vi "sort channels for specific data types.vi"(8 "error in (no error)":errorcluster, 10 "data types":T1[](array[typedef]), 11 "channels in":refnum<class "TBM channel.lvclass">[](array[class])) -> (0 "error out":errorcluster, 3 "channels out":refnum<class "TBM channel.lvclass">[](array[class]))   [LabVIEW 2014, in "Shared Memory configuration.lvclass"]
uses:
  Shared Memory configuration.lvclass
  <vilib>/NI/Tag Bus/tag/Data Type.ctl
  <vilib>/NI/Tag Bus Module Framework/channel/TBM channel.lvclass
  <vilib>/NI/Tag Bus Module Framework/channel/channel classification.ctl
  <vilib>/NI/Tag Bus/tag/tag descriptor.lvclass
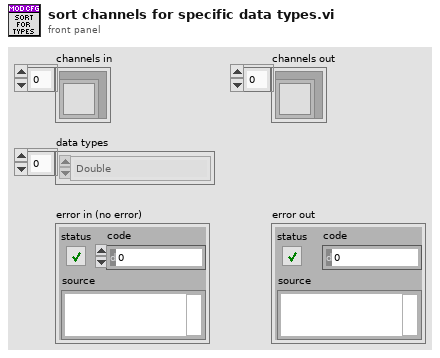
[diagram p1: front panel]
types:
  T1 = typedef "tag bus.lvlib/tag descriptor.lvclass/Data Type.ctl" = enum16{"Double", "Single", "I64", "I32", "I16", "I8", "U64", "U32", "U16", "U8", "Boolean", "String", "Array of Double", "Array of Single", "Array of I64", "Array of I32", "Array of I16", "Array of I8", "Array of U64", "Array of U32", "Array of U16", "Array of U8", "Array of Boolean", "Array of String"}
  T2 = typedef "TBM channel.lvclass/channel classification.ctl" = enum16{"input data", "output data", "processing parameter", "processing result"}
  T3 = cluster{"name":string, "system tag out":refnum<class "TBM channel.lvclass">}
  T4 = cluster{"name":string, "system tag out":refnum<class "TBM channel.lvclass">}[]
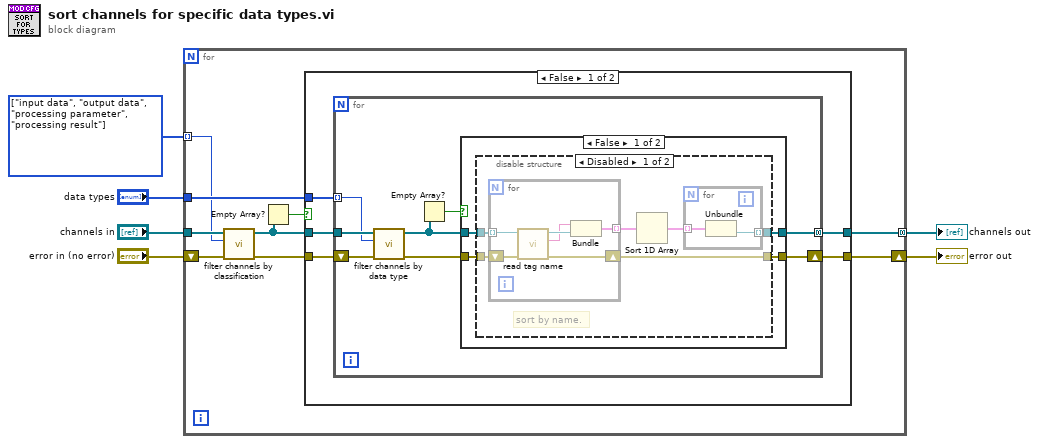
[diagram p0: block diagram]
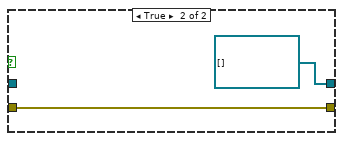
[diagram p3: hidden frame]
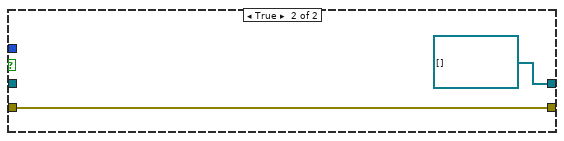
[diagram p4: hidden frame]
diagram:
  w2 = T2[] [enum."input data", enum."output data", enum."processing parameter", enum."processing result"] items=["input data", "output data", "processing parameter", "processing result"]
  n1 = for {
    tunnel: "data types" -> [w15]
    tunnel: "channels in" -> [w11]
    tunnel: [w14] -> w4 mode=concatenating
    tunnel: w2 -> [w9] mode=indexing
    shift-right: [w13] -> w5
    shift-left: "error in (no error)" -> [w12]
    n2 = call "filter channels by classification.vi"("error in (no error)"=w12, "channel classification"=w9, "channels in"=w11) -> ("error out"=w10:errorcluster, "filtered channels out"=w8:refnum<class "TBM channel.lvclass">[])  [unwired: 7 in]
    n3 = Empty Array?(array=w8) -> (empty?=w7:bool)
    n4 = case shown="False" w7 {
      tunnel: w15 -> [w20 _]
      tunnel: [w19 refnum<class "TBM channel.lvclass">[] []] -> w14
      tunnel: [w18 w52] -> w13
      tunnel: w10 -> [w17 w52]
      tunnel: w8 -> [w16 _]
      frame False {
        n5 = for {
          tunnel: w20 -> [w23] mode=indexing
          tunnel: [w27] -> w19 mode=concatenating
          shift-right: [w28] -> w18
          shift-left: w17 -> [w25]
          tunnel: w16 -> [w24]
          n6 = call "filter channels by data type.vi"("error in (no error)"=w25, "data type"=w23, "channels in"=w24) -> ("error out"=w21:errorcluster, "filtered channels out"=w22:refnum<class "TBM channel.lvclass">[])  [unwired: 7 in]
          n7 = Empty Array?(array=w22) -> (empty?=w26:bool)
          n8 = case shown="False" w26 {
            tunnel: [w32 w50] -> w28
            tunnel: [w31 refnum<class "TBM channel.lvclass">[] []] -> w27
            tunnel: w21 -> [w30 w50]
            tunnel: w22 -> [w29 _]
            frame False {
              n9 = disable-structure shown="Disabled" {
                disable-tunnel: [w38 w47] -> w32
                disable-tunnel: [w37 w48] -> w31
                disable-tunnel: w30 -> [w36 w47]
                disable-tunnel: w29 -> [w35 w48]
                frame Disabled {
                  # "sort by name."
                  n10 = for {
                    tunnel: w35 -> [w41] mode=indexing
                    shift-right: [w45] -> w38
                    shift-left: w36 -> [w46]
                    tunnel: [w42] -> w34 mode=indexing
                    n11 = call <vilib>:"read tag name.vi"("error in"=w46, "system tag in"=w41) -> ("error out"=w45:errorcluster, "name"=w43:string, "system tag out"=w44:refnum<class "TBM channel.lvclass">)  [unwired: 7 in]
                    n12 = Bundle("name"=w43, "system tag out"=w44) -> (w42:T3)  [unwired: 1 in]
                  }
                  n13 = Sort 1D Array(array=w34) -> (sorted array=w33:T4)
                  n14 = for {
                    tunnel: w33 -> [w40] mode=indexing
                    tunnel: [w39] -> w37 mode=indexing
                    n15 = Unbundle(w40) -> ("system tag out"=w39:refnum<class "TBM channel.lvclass">)  [unwired: 1 out]
                  }
                }
                frame Enabled {
                }
              }
            }
            frame True {
            }
          }
        }
      }
      frame True {
      }
    }
  }
  "error out" <- w5
  "channels out" <- w4
